vi "SMBUS Block Process Call.vi"(0 "DevIndex":i32, 1 "pWriteData":u8[](array[numeric])=array[4097 elements], 2 "pReadCount":i32, 5 "IICIndex":i32, 7 "SlaveAddr":i16, 9 "CommandCode":u8, 12 "WriteCount":i32, 13 "WithPEC":u8) -> (4 "pReadData":u8[](array[numeric]), 6 "pReadCount out":i32, 8 "function return":i32)   [LabVIEW 2010, in "usb2iic.lvlib"]
doc: "int WINAPI SMBUS_BlockProcessCall(int DevIndex,int IICIndex,short SlaveAddr,unsigned char CommandCode, unsigned char *pWriteData,int WriteCount, unsigned char *pReadData,int *pReadCount,unsigned char WithPEC);"
uses:
  usb2iic.lvlib
  USB2XXX.dll
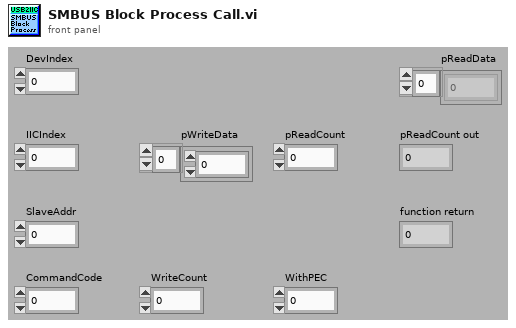
[diagram p1: front panel]
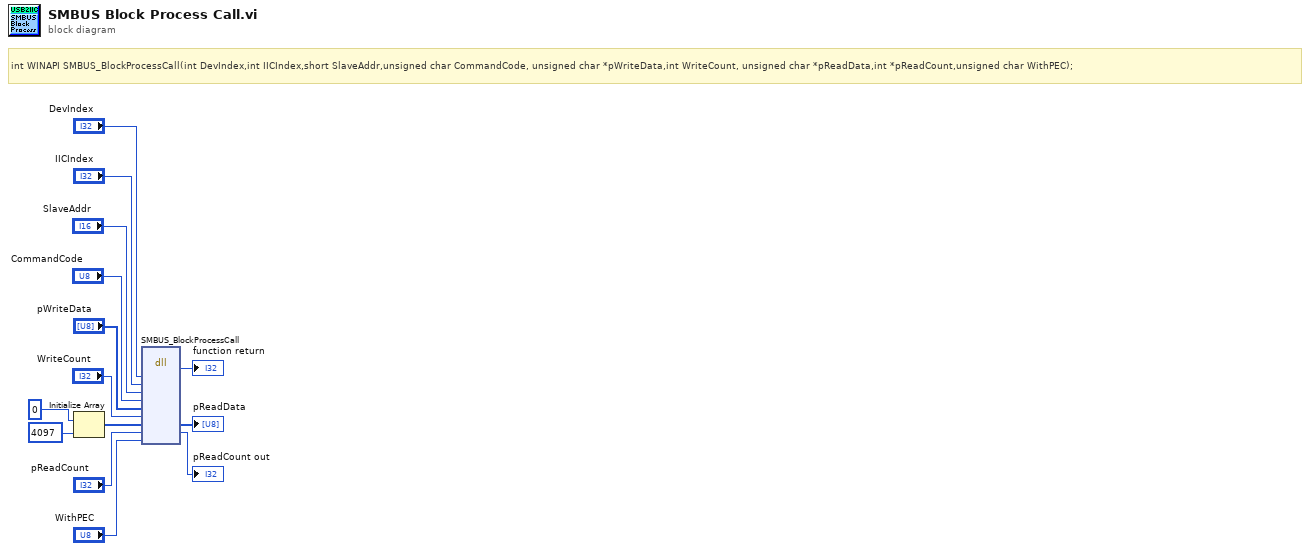
[diagram p0: block diagram]
diagram:
  # "int WINAPI SMBUS_BlockProcessCall(int DevIndex,int IICIndex,short SlaveAddr,unsigned char CommandCode, unsigned char *pWriteData,int WriteCount, unsigned char *pReadData,int *pReadCount,unsigned char WithPEC);"
  n1 = Initialize Array(u8 0 ("element"), 4097 ("dimension size")) -> (w7:u8[])
  n2 = dll-call lib="G:/OtherWork/USB2XXX_Example/trunk/Labview/PublicFiles/usb2iic/USB2XXX.*" fn="SMBUS_BlockProcessCall"("DevIndex"="DevIndex", "IICIndex"="IICIndex", "SlaveAddr"="SlaveAddr", "CommandCode"="CommandCode", "pWriteData"="pWriteData", "WriteCount"="WriteCount", "pReadData"=w7, "pReadCount"="pReadCount", "WithPEC"="WithPEC") -> (→"function return":i32, "pReadData"=→"pReadData":u8[], "pReadCount"=→"pReadCount out":i32)  [unwired: 10 in, 2 out]
